vi "check_set_ID_response.vi"(4 "IDN string parsing regex\n\"(Rohde-Schwarz|Rohde&Schwarz|HAMEG),([^,]+),([^,]+),([^,]+)\"":string="(Rohde-Schwarz|Rohde&Schwarz|HAMEG),([^,]+),([^,]+),([^,]+)", 6 "Supported instruments in":string[](array[string]), 7 "Error if ID Query check fails":bool, 8 "error in":errorcluster caption="error in (no error)", 9 "Aliases in (\"\")":string, 10 "IDN string in":string, 11 "VISA resource name":refnum<visa-resource-name>) -> (0 "error out":errorcluster, 1 "Instrument supported":bool, 2 "Instrument type out":string, 3 "VISA resource name out":refnum<visa-resource-name>)   [LabVIEW 2020, in "Rohde&Schwarz RTx Oscilloscopes.lvlib" / "rsidr_core.lvlib"]
uses:
  rsidr_core.lvlib
  type_Error_Codes.ctl
  _type_Operation_Fgv_Session.ctl
  Match Regular Expression.xnode
panel:
  out "Alias used":bool
  # "Aliases expression can be used\nfor mapping purposes. Syntax:\n<physical device1_Regex> -> <alias1>\\n\n<physical device2_Regex> -> <alias2>\\n\n\nExamples:\nto have FSWP-33 to be treated as FSVR:\n^FSWP-33$ -> FSVR\nany FSVA to be treated as FSV:\n^FSVA-[0-9]+$ -> FSV"
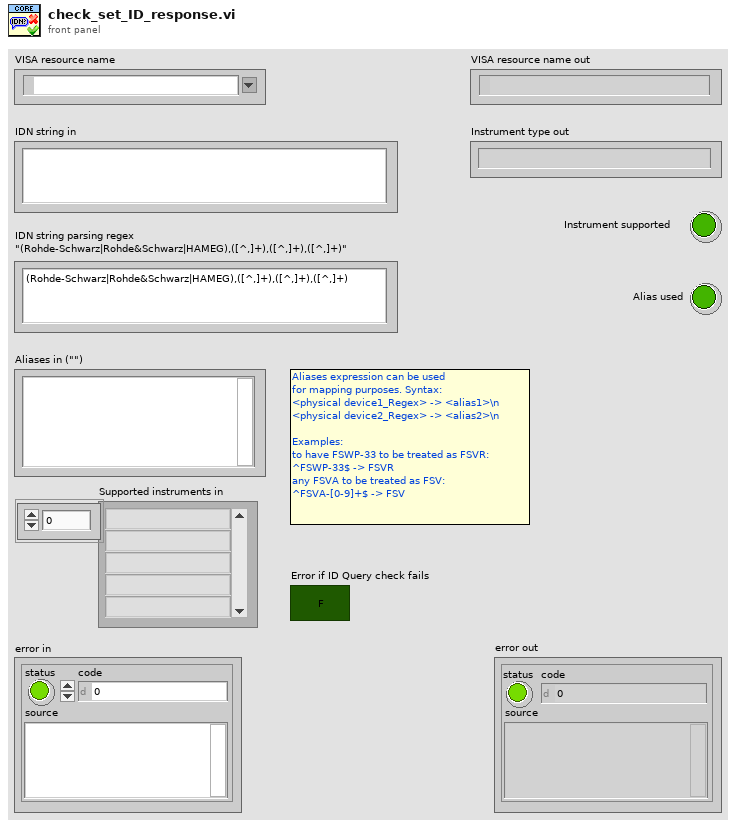
[diagram p1: front panel]
types:
  T1 = typedef "Rohde&Schwarz RTx Oscilloscopes.lvlib/rsidr_core.lvlib/_type_Operation_Fgv_Session.ctl" = enum16{"Initialize", "GetData", "SetData", "Clear", "GetSessionIx"}
  T2 = typedef "Rohde&Schwarz RTx Oscilloscopes.lvlib/rsidr_core.lvlib/type_Error_Codes.ctl" = enum16{"No_error", "VISA_err_ResourceNotFound", "VISA_err_Timeout", "VISA_warn_MoreDataAvailable", "RS_err_MissingCallback", "RS_err_InvalidAttribute", "RS_err_InvalidValue", "RS_err_UnknownResource", "RS_err_AlreadyInitialized", "RS_err_InstrumentStatus", "RS_err_BadRepCapName", "RS_err_TypesMismatch", "RS_err_ValueNotSupported", "RS_err_InvalidRngTable", "RS_err_IDqueryFail", "RS_err_UnexpResponse", "VISA_warn_ConfigNotLoaded", "RS_err_AttributeNotReadable", "RS_err_AttributeNotWritable", "RS_err_InstrumentType", "RS_err_InstrumentOption", "VISA_err_InvalidSize", "RS_err_ReliabilityIndicator", "VISA_warn_UnknownStatus", "VISA_warn_TermCharRead", "VISA_err_IO_error", "RS_err_FunctionNotSupported", "VISA_warn_QueueEmpty"}
  T3 = typedef "Rohde&Schwarz RTx Oscilloscopes.lvlib/rsidr_core.lvlib/type_Session_Data.ctl" = cluster{"IDN string":string, "Instrument FW":string, "Instr type":string, "Instr type for err. msg.":string, "Installed Options":string[], "Ignore Error Messages":string, "Logging params":variant, "OPC Timeout":i32, "VISA Timeout":i32, "STB Poll VISA Timeout":i32, "Additional Flags":i32, "Wait Before Read":i32, "Wait Before Write":i32, "Option String Flags":i32, "IO Segment Size":i64, "VISA Access Mode":T4, "Interface Type":T5, "OPC Wait Mode":T6, "Bin Float Number  Format":T7, "Bin Integer Number Format":T8, "Simulate":bool, "VXIcapable":bool, "Duplicate Session":bool, "Add LF to Write":bool, "Logging":bool, "Fast Sweep":bool, "Query Instrument Status":bool, "Check Range":bool, "Check Options":bool, "OPC-sync Attr Writes":bool, "OPC-sync Attr Queries":bool}
  T4 = typedef "Rohde&Schwarz RTx Oscilloscopes.lvlib/rsidr_core.lvlib/type_VisaAccessMode.ctl" = u16
  T5 = typedef "Rohde&Schwarz RTx Oscilloscopes.lvlib/rsidr_core.lvlib/type_InterfaceType.ctl" = enum16{"Unknown", "GPIB", "VXI", "GPIB_VXI", "ASRL", "PXI", "TCPIP", "USB", "SOCKET"}
  T6 = typedef "Rohde&Schwarz RTx Oscilloscopes.lvlib/rsidr_core.lvlib/type_OPC_Wait_Mode.ctl" = enum16{"STBpolling", "STBpollingSlow", "STBpollingSuperSlow", "ServiceRequest", "OPCquery"}
  T7 = typedef "Rohde&Schwarz RTx Oscilloscopes.lvlib/rsidr_core.lvlib/type_Binary_Float_Number_Format.ctl" = enum16{"Float_4_Bytes_Swapped", "Float_4_Bytes", "Double_8_Bytes_Swapped", "Double_8_Bytes"}
  T8 = typedef "Rohde&Schwarz RTx Oscilloscopes.lvlib/rsidr_core.lvlib/type_Binary_Integer_Number_Format.ctl" = enum16{"Int32_4_Bytes_Swapped", "Int32_4 Bytes", "Int16_2_Bytes_Swapped", "Int16_2_Bytes"}
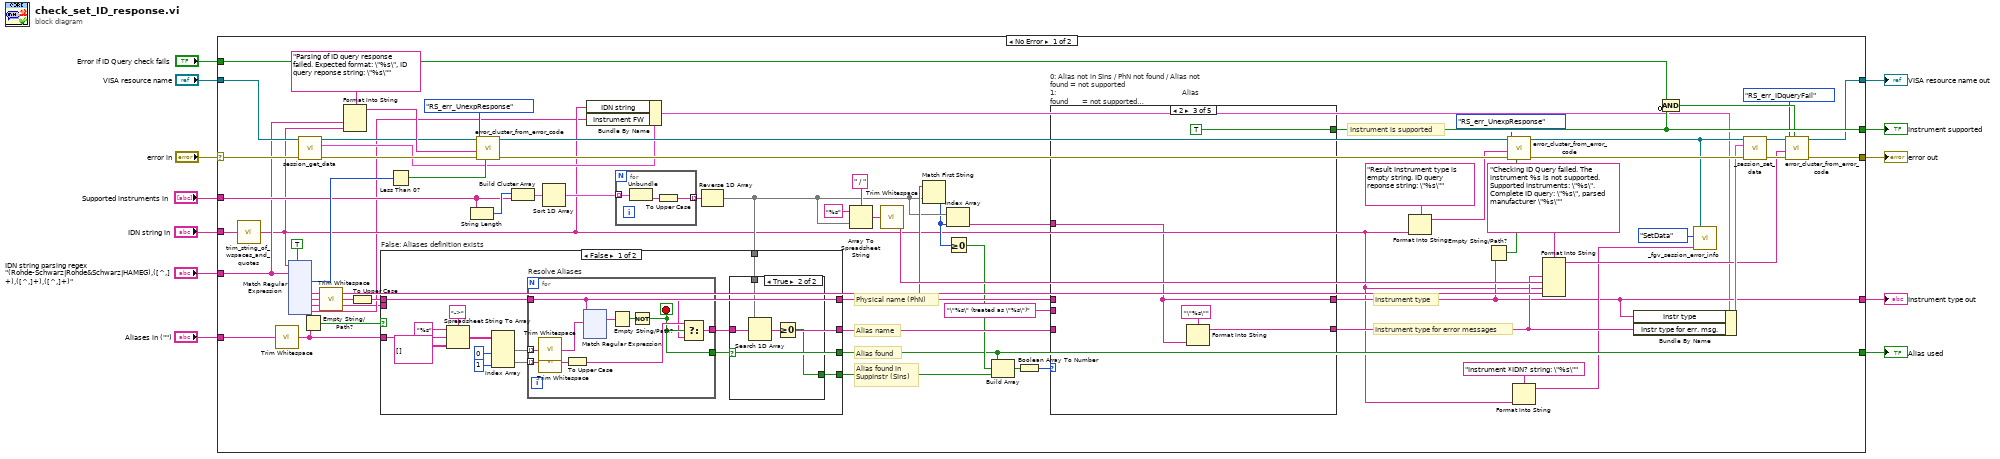
[diagram p0: block diagram]
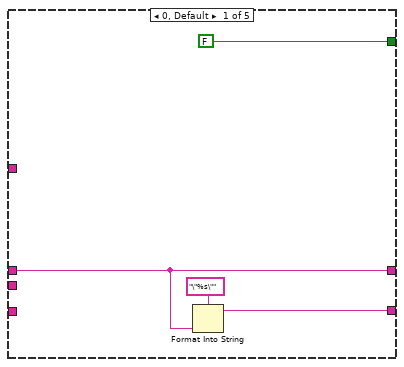
[diagram p4: hidden frame]
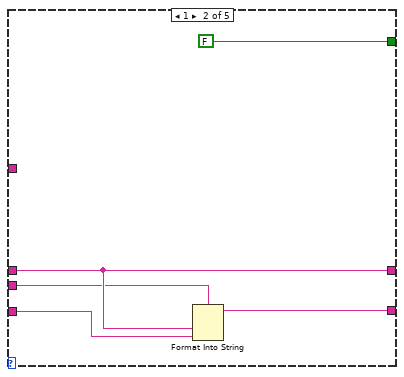
[diagram p5: hidden frame]
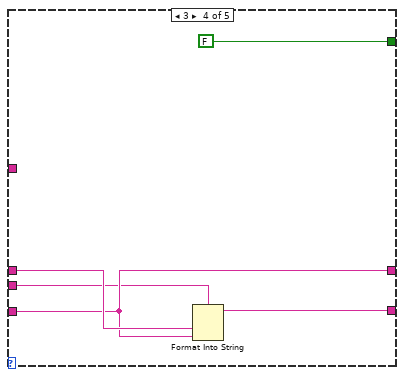
[diagram p6: hidden frame]
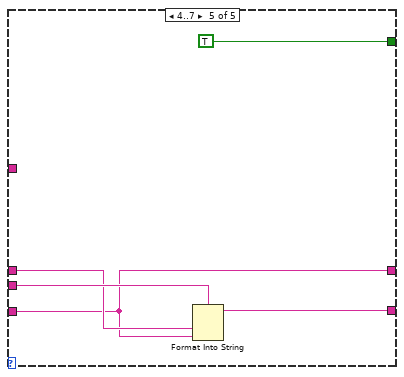
[diagram p7: hidden frame]
diagram:
  n1 = case shown="No Error" "error in" {
    selector: "error in" -> [w78 w364]
    tunnel: [w80 w364] -> w12
    tunnel: [w21 _] -> w10
    tunnel: [w79 _] -> w9
    tunnel: "VISA resource name" -> [w76 w363]
    tunnel: [w44 w363] -> w7
    tunnel: [w31 _] -> w6
    tunnel: "Error if ID Query check fails" -> [w27 _]
    tunnel: "Supported instruments in" -> [w26 _]
    tunnel: "IDN string in" -> [w18 _]
    tunnel: "IDN string parsing regex\n\"(Rohde-Schwarz|Rohde&Schwarz|HAMEG),([^,]+),([^,]+),([^,]+)\"" -> [w25 _]
    tunnel: "Aliases in (\"\")" -> [w24 _]
    frame No Error {
      # "Alias found in\nSuppInstr (SIns)"
      # "Alias found"
      # "Instrument is supported"
      # "Instrument type for error messages"
      # "Instrument type"
      # "Physical name (PhN)"
      # "Alias name"
      n2 = call "trim_string_of_wspaces_and_quotes.vi"("String in"=w18) -> ("String out"=w17:string)  [unwired: 4 in]
      n3 = call "Trim Whitespace.vi"("string"=w24) -> ("trimmed string"=w64:string)  [unwired: 1 in]
      n4 = xnode ("Match Regular Expression")("input string"=w17, "regular expression"=w25, "ignore case? (F)"=TRUE) -> ("offset past match"=w62:i32, "submatch 1"=w68:string, "submatch 2"=w35:string, "submatch 3"=w15:string, "submatch 4"=w16:string)  [unwired: 3 in, 4 out]
      n5 = call "session_get_data.vi"("error in"=w78, "VISA resource name"=w76) -> ("error out"=w77:errorcluster, "Session User Data out"=w20:T3, "VISA resource name out"=w48:refnum<visa-resource-name>)  [unwired: 6 in, 1 out]
      n6 = Empty String/Path?(string/path=w64) -> (empty?=w63:bool)
      n7 = call "Trim Whitespace.vi"("string"=w35) -> ("trimmed string"=w23:string)  [unwired: 1 in]
      n8 = Format Into String(format string="Parsing of ID query response failed. Expected format: \"%s\", ID query reponse string: \"%s\"", w25, w17) -> (resulting string=w50:string)  [unwired: 2 in, 1 out]
      n9 = To Upper Case(1:w23) -> (0:w22:string)
      n10 = Less Than 0?(x=w62) -> (x < 0?=w61:bool)
      n11 = String Length(string=w26) -> (length=w65:i32[])
      n12 = call "error_cluster_from_error_code.vi"("Error Creation Enabled (True)"=w61, "error in"=w77, "Error Message (\"\")"=w50, "Error Enum in"=type_Error_Codes."RS_err_UnexpResponse", "VISA resource name"=w48) -> ("error out"=w59:errorcluster, "VISA resource name out"=w49:refnum<visa-resource-name>)  [unwired: 5 in]
      n13 = Build Cluster Array ("Index & Bundle Cluster Array")(w65, w26) -> (w70:cluster{"Element":i32, "Element":string}[])
      n14 = Sort 1D Array(array=w70) -> (sorted array=w69:cluster{"Element":i32, "Element":string}[])
      n15 = Bundle By Name(cluster=w20, "IDN string"=w17, "Instrument FW"=w16) -> (w19:T3)
      n16 = for {
        tunnel: w69 -> [w223] mode=indexing
        tunnel: [w221] -> w51 mode=indexing
        n17 = Unbundle(w223) -> ("Element"=w222:string)  [unwired: 1 out]
        n18 = To Upper Case(1:w222) -> (0:w221:string)
      }
      n19 = Reverse 1D Array(array=w51) -> (reversed array=w37:string[])
      n20 = case "False: Aliases definition exists" shown="False" w63 {
        tunnel: w22 -> [w81 w220]
        tunnel: [w83 _] -> w71
        tunnel: [w85 _] -> w31
        tunnel: w64 -> [w89 _]
        tunnel: [w81 w220] -> w38
        tunnel: w37 -> [w84 _]
        tunnel: [w82 _] -> w33
        tunnel: w15 -> [_ _]
        frame False {
          n21 = Spreadsheet String To Array(delimiter (Tab)="->", format string="%s", spreadsheet string=w89, array type (2D Dbl)=string[][] [] ("Array")) -> (array=w91:string[][])
          n22 = Index Array(array=w91, index (col) #1=0 ("index (row)"), index (col) #2=1 ("index (row)")) -> (element #1=w86:string[], element #2=w90:string[])  [unwired: 2 in]
          n23 = for "Resolve Aliases" {
            tunnel: w86 -> [w108] mode=indexing
            tunnel: w90 -> [w107] mode=indexing
            tunnel: [w105] -> w83
            tunnel: [w102] -> w85
            tunnel: w81 -> [w101]
            stop <- w102 stop-if-true
            n24 = call "Trim Whitespace.vi"("string"=w108) -> ("trimmed string"=w100:string)  [unwired: 1 in]
            n25 = call "Trim Whitespace.vi"("string"=w107) -> ("trimmed string"=w106:string)  [unwired: 1 in]
            n26 = To Upper Case(1:w106) -> (0:w104:string)
            n27 = xnode "Match Regular Expression"("input string"=w101, "regular expression"=w100) -> ("whole match"=w99:string)  [unwired: 4 in, 4 out]
            n28 = Empty String/Path?(string/path=w99) -> (empty?=w103:bool)
            n29 = Not(x=w103) -> (.not. x?=w102:bool)
            n30 = Select(t=w104, s=w102, f=w101) -> (s? t:f=w105:string)
          }
          n31 = case shown="True" w85 {
            tunnel: w84 -> [_ w98]
            tunnel: w83 -> [_ w97]
            tunnel: [_ w95] -> w82
            frame False {
            }
            frame True {
              n32 = Search 1D Array(1D array=w98, element=w97) -> (index of element=w96:i32)  [unwired: 1 in]
              n33 = Greater Or Equal To 0?(x=w96) -> (x >= 0?=w95:bool)
            }
          }
        }
        frame True {
        }
      }
      n34 = Array To Spreadsheet String(delimiter (Tab)=" / ", array=w37, 3:"%s" ("format string")) -> (spreadsheet string=w74:string)
      n35 = call "Trim Whitespace.vi"("string"=w74) -> ("trimmed string"=w57:string)  [unwired: 1 in]
      n36 = Match First String(2:w37, 3:w38) -> (0:w36:i32)  [unwired: 1 out]
      n37 = Index Array(array=w37, index=w36) -> (element=w32:string)
      n38 = Greater Or Equal To 0?(x=w36) -> (x >= 0?=w34:bool)
      n39 = Build Array(w31, w34, w33) -> (w40:bool[])
      n40 = Boolean Array To Number(Boolean array=w40) -> (number=w39:u32)
      n41 = case "0: Alias not in SIns / PhN not found / Alias not found = not supported\n1:                                                               Alias found       = not supported\n2:                                 PhN found                                      = supported PhN\n3: Alias not in SIns    PhN found           Alias found       = not supported\n4..7: Alias in SIns                                                                 = supported allias" shown="2" w39 {
        tunnel: w71 -> [_ w229 _ w238 w242]
        tunnel: w38 -> [w225 w230 _ w239 w243]
        tunnel: [w225 w230 w233 w238 w242] -> w21
        tunnel: [w224 w231 w234 w240 w245] -> w54
        tunnel: [FALSE FALSE TRUE FALSE TRUE] -> w79
        tunnel: w32 -> [_ _ w233 _ _]
        tunnel: "\"%s\" (treated as \"%s\")" ("format string") -> [_ w228 _ w237 w244]
        frame 0, Default {
          n42 = Format Into String(format string="\"%s\"", w225) -> (resulting string=w224:string)  [unwired: 2 in, 1 out]
        }
        frame 1 {
          n43 = Format Into String(format string=w228, w230, w229) -> (resulting string=w231:string)  [unwired: 2 in, 1 out]
        }
        frame 2 {
          n44 = Format Into String(format string="\"%s\"", w233) -> (resulting string=w234:string)  [unwired: 2 in, 1 out]
        }
        frame 3 {
          n45 = Format Into String(format string=w237, w239, w238) -> (resulting string=w240:string)  [unwired: 2 in, 1 out]
        }
        frame 4..7 {
          n46 = Format Into String(format string=w244, w243, w242) -> (resulting string=w245:string)  [unwired: 2 in, 1 out]
        }
      }
      n47 = Format Into String(format string="Result Instrument type is empty string. ID query reponse string: \"%s\"", w17) -> (resulting string=w47:string)  [unwired: 2 in, 1 out]
      n48 = Empty String/Path?(string/path=w21) -> (empty?=w58:bool)
      n49 = call "error_cluster_from_error_code.vi"("Error Creation Enabled (True)"=w58, "error in"=w59, "Error Message (\"\")"=w47, "Error Enum in"=type_Error_Codes."RS_err_UnexpResponse", "VISA resource name"=w49) -> ("error out"=w53:errorcluster, "VISA resource name out"=w30:refnum<visa-resource-name>)  [unwired: 5 in]
      n50 = Format Into String(format string="Instrument *IDN? string: \"%s\"", w17) -> (resulting string=w28:string)  [unwired: 2 in, 1 out]
      n51 = Format Into String(format string="Checking ID Query failed. The instrument %s is not supported. Supported instruments: \"%s\". Complete ID query: \"%s\", parsed manufacturer \"%s\"", w54, w57, w17, w68) -> (resulting string=w43:string)  [unwired: 2 in, 1 out]
      n52 = Bundle By Name(cluster=w19, "Instr type"=w21, "Instr type for err. msg."=w54) -> (w52:T3)
      n53 = Compound Arithmetic op=AND(w27, invert w79) -> (w66:bool)
      n54 = call "_fgv_session_error_info.vi"("Session Error Info in (\"\")"=w28, "Operation"=_type_Operation_Fgv_Session."SetData", "Session in"=w30) -> ()  [unwired: 3 in, 2 out]
      n55 = call "_session_set_data.vi"("error in"=w53, "Session User Data in"=w52, "VISA resource name"=w30) -> ("error out"=w55:errorcluster, "VISA resource name out"=w45:refnum<visa-resource-name>)  [unwired: 7 in]
      n56 = call "error_cluster_from_error_code.vi"("Error Creation Enabled (True)"=w66, "error in"=w55, "Error Message (\"\")"=w43, "Error Enum in"=type_Error_Codes."RS_err_IDqueryFail", "VISA resource name"=w45) -> ("error out"=w80:errorcluster, "VISA resource name out"=w44:refnum<visa-resource-name>)  [unwired: 5 in]
    }
    frame Error {
    }
  }
  "VISA resource name out" <- w7
  "error out" <- w12
  "Instrument type out" <- w10
  "Instrument supported" <- w9
  "Alias used" <- w6
